vi "CalculateAreaOfFirstPeakofSizeDistribution.vi"(1 "Extinction ExtinctionUncertainity Size parameter and Number ofS sizes":T1={"Extinction"=[], "Extinction Uncertainty"=[], "Size parameters"=[], "Number ofSizes"=0.0, "GeometricCrossSection"=[], "Wave Length"=0.0, "SMPS Sizes"=[], "Concentration"=[], "Double Charge Correction"=FALSE, "Extincation Factor"=1.0, "Diameter Factor"=1.0, "Diameter Offset"=0.0, "Extinction Factor Flag"=FALSE, "Diameter Factor Flag"=FALSE, "Diameter Offset Flag"=FALSE, "Sizes"=[], "ExtinctionOrAbsorptionOrScattering"=0, "Convergence Strength"=enum."Weak"} {"ExtinctionOrAbsorptionOrScattering" scale=0.0..2.0}) -> (0 "Area of First peak":dbl[](array[numeric]))   [LabVIEW 2013]
uses:
  BaesDataTypeDefinition.ctl
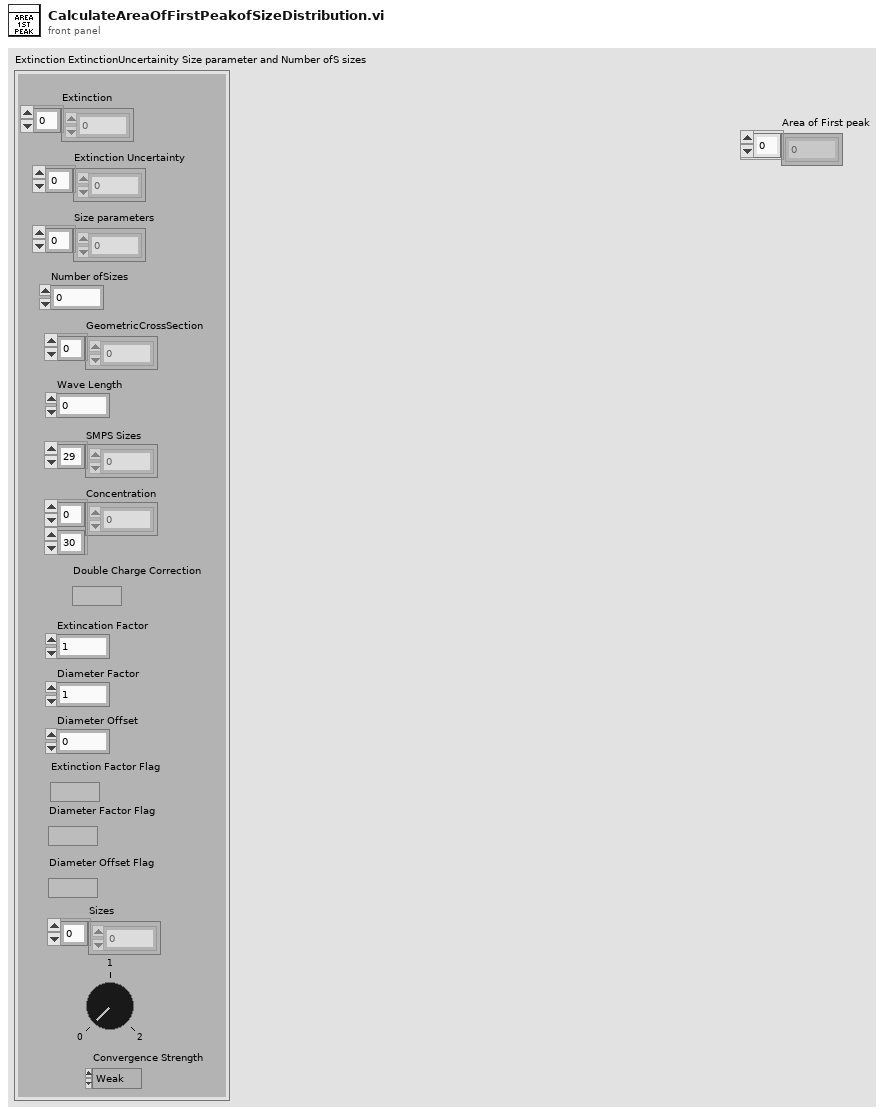
[diagram p1: front panel]
types:
  T1 = typedef "BaesDataTypeDefinition.ctl" = cluster{"Extinction":dbl[], "Extinction Uncertainty":dbl[], "Size parameters":dbl[], "Number ofSizes":dbl, "GeometricCrossSection":dbl[], "Wave Length":dbl, "SMPS Sizes":dbl[], "Concentration":dbl[][], "Double Charge Correction":bool, "Extincation Factor":dbl, "Diameter Factor":dbl, "Diameter Offset":dbl, "Extinction Factor Flag":bool, "Diameter Factor Flag":bool, "Diameter Offset Flag":bool, "Sizes":dbl[], "ExtinctionOrAbsorptionOrScattering":i8, "Convergence Strength":enum16{"Weak", "Medium", "Strong"}}
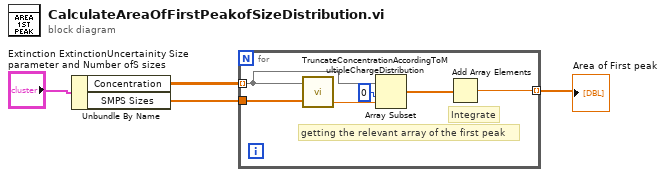
[diagram p0: block diagram]
diagram:
  n1 = Unbundle By Name("Extinction ExtinctionUncertainity Size parameter and Number ofS sizes") -> ("Concentration"=w3:dbl[][], "SMPS Sizes"=w2:dbl[])
  n2 = for {
    tunnel: w3 -> [w9] mode=indexing
    tunnel: w2 -> [w10]
    tunnel: [w5] -> w1 mode=indexing
    # "Integrate"
    # "getting the relevant array of the first peak"
    n3 = call "TruncateConcentrationAccordingToMultipleChargeDistribution.vi"("Concentration"=w9, "Sizes"=w10) -> ("Location"=w7:dbl)  [unwired: 2 out]
    n4 = Array Subset(array=w9, index=0, length=w7) -> (w6:dbl[])
    n5 = Add Array Elements(numeric array=w6) -> (sum=w5:dbl)
  }
  "Area of First peak" <- w1
